vi "Test TCRS Temperature At Initial Value if Heater Disabled.vi"(8 "error in (no error)":errorcluster, 11 "Thermal Chamber Response Simlator Test In":refnum<class "Thermal Chamber Response Simlator Test.lvclass">) -> (0 "error out":errorcluster, 3 "Thermal Chamber Response Simlator Test Out":refnum<class "Thermal Chamber Response Simlator Test.lvclass">)   [LabVIEW 2020, in "Thermal Chamber Response Simlator Test.lvclass"]
uses:
  Thermal Chamber Response Simlator Test.lvclass
  C:/Program Files (x86)/National Instruments/LabVIEW 2020/vi.lib/Astemes/LUnit/Test Case.lvclass
  Thermal Chamber Response Simlator/Thermal Chamber Response Simlator.lvclass
  Thermal Chamber Response Simlator/Thermal Chamber Response Simlator.lvclass/Thermal Chamber Response Simlator.ctl
  <vilib>/Astemes/LUnit/Test Case.lvclass/Test Case.ctl
  <vilib>/Astemes/LUnit/Palette/Pass If Equal.vi/cbf50e99-f124-4847-863a-8e9794d3dede.vi
  <vilib>/Astemes/LUnit/Palette/Pass.vi
  <vilib>/Astemes/LUnit/Palette/Fail.vi
  <vilib>/Astemes/LUnit/Compare Variants.vi
  <vilib>/Astemes/LUnit/Describe Comparison.vi
  <vilib>/Astemes/LUnit/Set Assertion Type.vi
  <vilib>/Astemes/LUnit/Add test result.vi
  <vilib>/Astemes/LUnit/Variant to string.vi
  <vilib>/Astemes/LUnit/LUnit Record Assertion Result.vi
  <vilib>/Astemes/LUnit/LUnit Aggregate Assertion Results.vi
  <vilib>/Astemes/LUnit/Method Result/LUnit Merge Status.vi
  <vilib>/Astemes/LUnit/LUnit Concatenate result strings.vi
  Thermal Chamber Response Simlator/Private/Get Current Time if Not Set.vi
  <vilib>/Utility/Data Type/Get Type Information.vi
  <vilib>/Utility/LVClass/Get LV Class Name.vi
  <vilib>/Astemes/LUnit/Test Case.lvclass
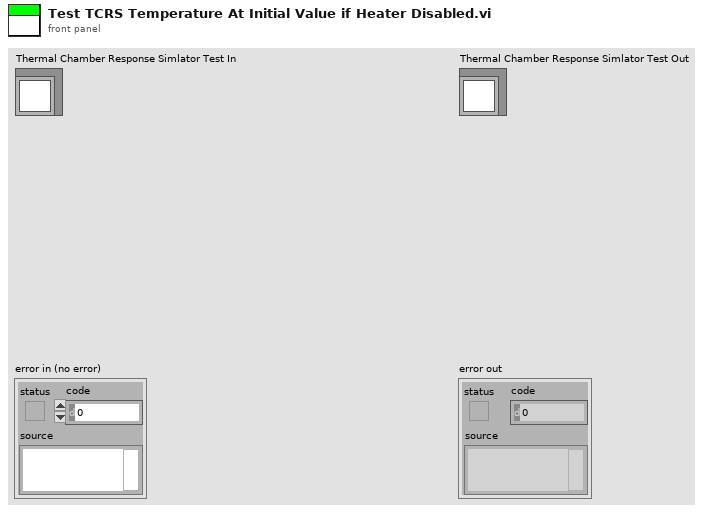
[diagram p1: front panel]
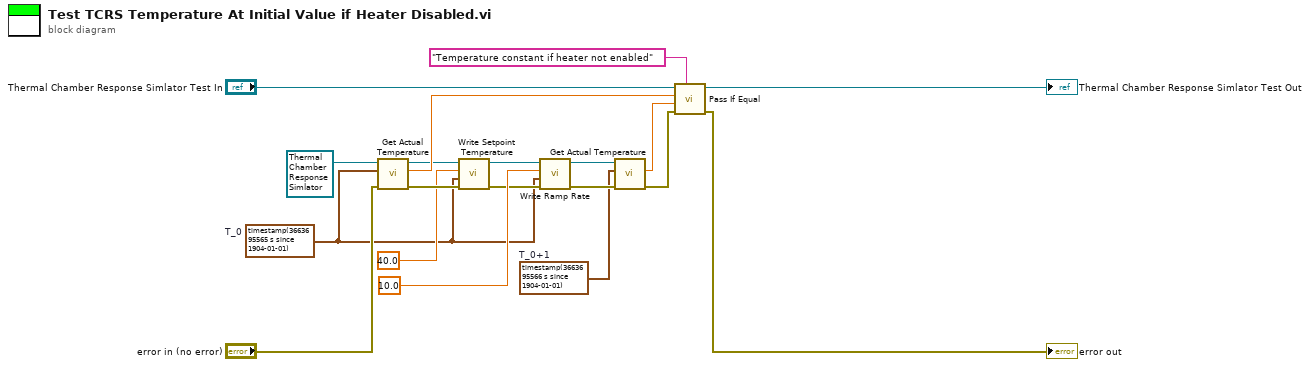
[diagram p0: block diagram]
diagram:
  w13 = timestamp(3663695566 s since 1904-01-01)  # T_0+1
  w1 = timestamp(3663695565 s since 1904-01-01)  # T_0
  n1 = call "Get Actual Temperature.vi"("error in (no error)"="error in (no error)", "Time Stamp"=w1, "Thermal Chamber Response Simlator In"=refnum<class "Thermal Chamber Response Simlator.lvclass"> refnum ("Thermal Chamber Response Simlator.lvclass")) -> ("error out"=w17:errorcluster, "Actual Temperature [degC]"=w9:dbl, "Thermal Chamber Response Simlator Out"=w4:refnum<class "Thermal Chamber Response Simlator.lvclass">)  [unwired: 6 in]
  n2 = call "Write Setpoint Temperature.vi"("error in (no error)"=w17, "Update Time"=w1, "Setpoint Temperature [degC]"=40.0, "Thermal Chamber Response Simlator In"=w4) -> ("error out"=w5:errorcluster, "Thermal Chamber Response Simlator Out"=w3:refnum<class "Thermal Chamber Response Simlator.lvclass">)  [unwired: 6 in]
  n3 = call "Write Ramp Rate.vi"("error in (no error)"=w5, "Time Stamp"=w1, "Ramp Rate [degC/s]"=10.0, "Thermal Chamber Response Simlator In"=w3) -> ("error out"=w14:errorcluster, "Thermal Chamber Response Simlator Out"=w15:refnum<class "Thermal Chamber Response Simlator.lvclass">)  [unwired: 6 in]
  n4 = call "Get Actual Temperature.vi"("error in (no error)"=w14, "Time Stamp"=w13, "Thermal Chamber Response Simlator In"=w15) -> ("error out"=w11:errorcluster, "Actual Temperature [degC]"=w10:dbl)  [unwired: 6 in, 1 out]
  n5 = call <vilib>:"Pass If Equal.vi"("Description"="Temperature constant if heater not enabled", "error in (no error)"=w11, "Actual"=w10, "Expected"=w9, "LUnit Test Case In"="Thermal Chamber Response Simlator Test In") -> ("error out"=→"error out":errorcluster, "LUnit Test Case Out"=→"Thermal Chamber Response Simlator Test Out":refnum<class "Thermal Chamber Response Simlator Test.lvclass">)  [unwired: 5 in]
